vi "ReadBuffer.vi"(2 "Data type":T2(ring)=enum."I16", 5 "Pointer and BufferSize":u64[](array[numeric]), 7 "Offset":u64, 9 "Buffer size":i32, 11 "error in (no error)":errorcluster) -> (6 "Output Array":i16[](array[numeric]), 15 "error out":errorcluster)   [LabVIEW 2024]
uses:
  <vilib>/Utility/error.llb/DialogType.ctl
panel:
  in  "type of dialog (OK msg:1)":T1=4 items=["no dialog", "OK message", "continue or stop message", "OK message + warnings", "continue/stop + warnings"]
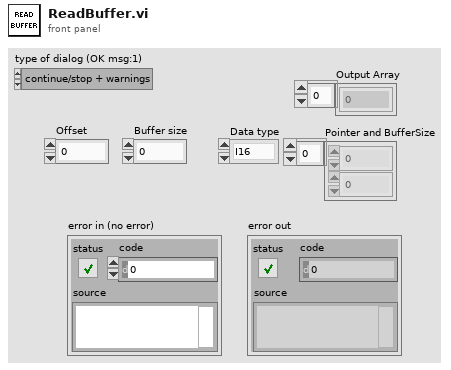
[diagram p1: front panel]
types:
  T1 = typedef "DialogType.ctl" = u16
  T2 = enum16{"U8", "I8", "U16", "I16", "U32", "I32", "U64", "I64"}
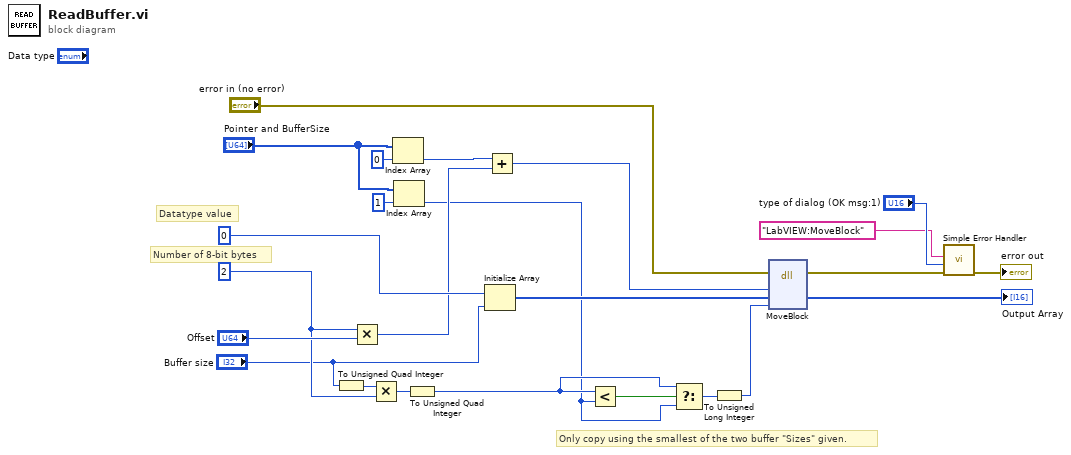
[diagram p0: block diagram]
diagram:
  w10 = u64 2 ("y")
  # "Number of 8-bit bytes"
  # "Datatype value"
  # "Only copy using the smallest of the two buffer \"Sizes\" given."
  n1 = To Unsigned Quad Integer(1:"Buffer size") -> (0:w9:u64)
  n2 = Multiply(x=w10, y="Offset") -> (x*y=w18:u64)
  n3 = Multiply(x=w9, y=w10) -> (x*y=w17:u64)
  n4 = Index Array(array="Pointer and BufferSize", index=0) -> (element=w20:u64)
  n5 = Index Array(array="Pointer and BufferSize", index=1) -> (element=w5:u64)
  n6 = To Unsigned Quad Integer(1:w17) -> (0:w12:u64)
  n7 = Initialize Array(i16 0 ("element"), "Buffer size") -> (w14:i16[])
  n8 = Add(x=w20, y=w18) -> (x+y=w15:u64)
  n9 = Less?(x=w12, y=w5) -> (x < y?=w11:bool)
  n10 = Select(t=w12, s=w11, f=w5) -> (s? t:f=w7:u64)
  n11 = To Unsigned Long Integer(number=w7) -> (unsigned 32bit integer=w6:u32)
  n12 = dll-call lib="LabVIEW" fn="MoveBlock"(error in="error in (no error)", "Source"=w15, "Destination"=w14, "Size"=w6) -> (error out=w2:errorcluster, "Destination"=→"Output Array":i16[])  [unwired: 5 in, 1 out]
  n13 = call <vilib>:"Simple Error Handler.vi"("error source (\" \")"="LabVIEW:MoveBlock", "type of dialog (OK msg:1)"="type of dialog (OK msg:1)", "error in (no error)"=w2) -> ("error out"=→"error out":errorcluster)  [unwired: 2 in, 4 out]
